vi "2_ExportDatatoExcel.vi"(8 "error in (no error)":errorcluster, 10 "Waveform Graph":waveform(dbl)[](graph), 11 "file path (IN)":path) -> (0 "error out":errorcluster, 3 "file path (OUT)":path)   [LabVIEW 2020]
uses:
  <vilib>/Utility/file.llb/Write Delimited Spreadsheet (string).vi
panel:
  out "Ch3 : Y":dbl[](array[numeric])
  out "Ch3 : appended array":string[](array[string])
  out "Ch1 : appended array":string[](array[string])
  out "Ch1 : Y":dbl[](array[numeric])
  out "dt":dbl
  out "Spread Sheet Display":string[][](array[string])
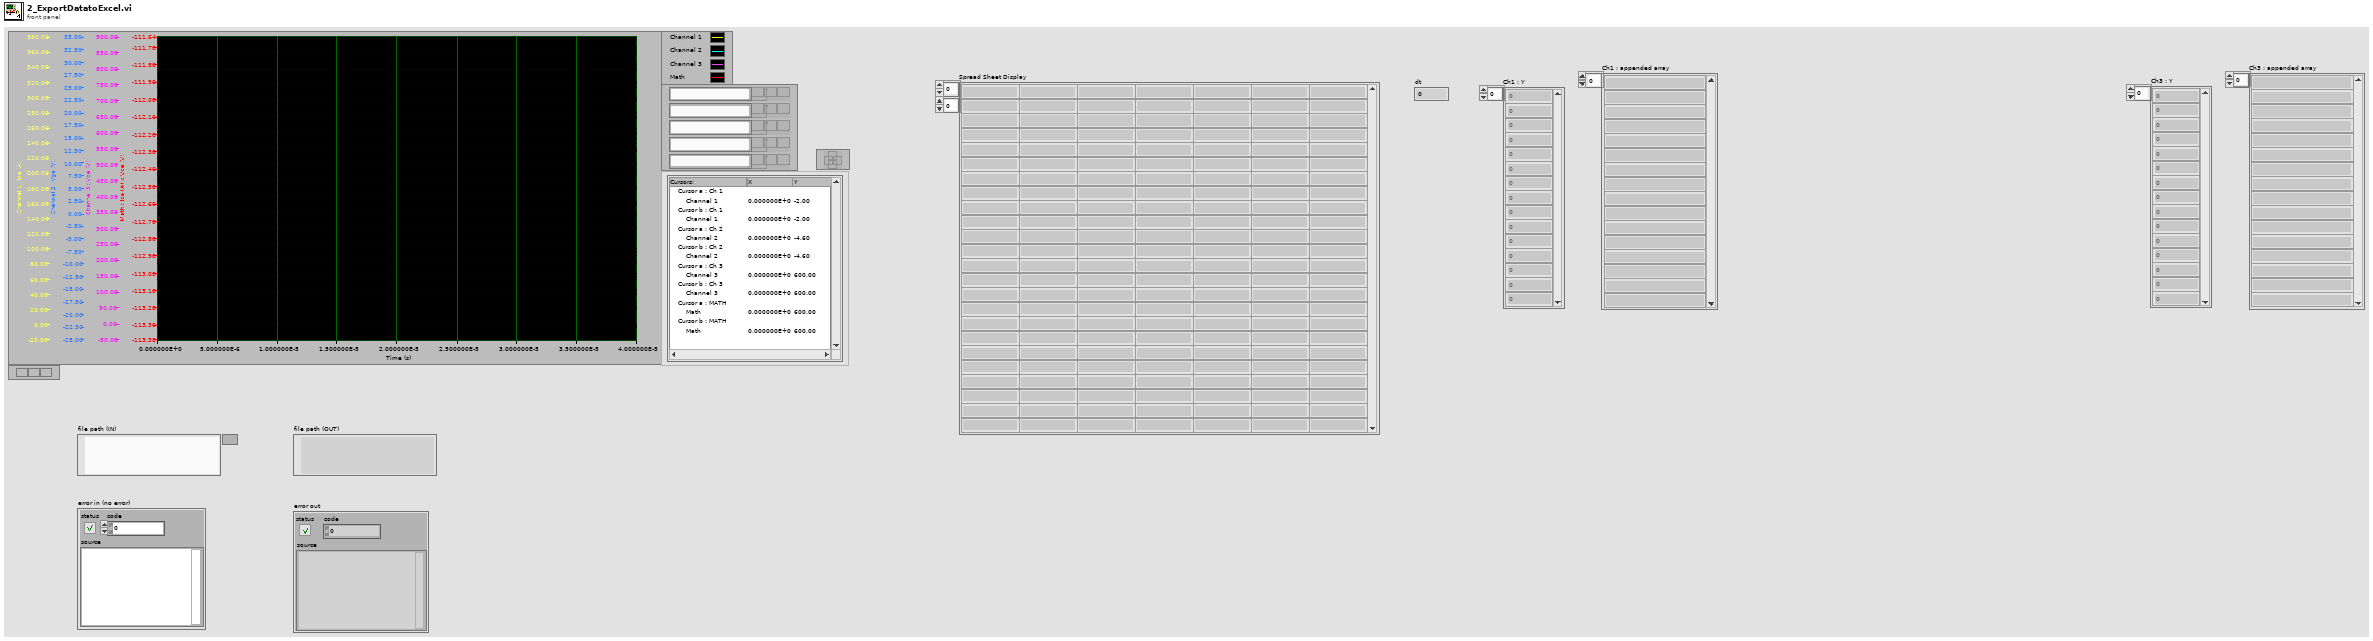
[diagram p1: front panel]
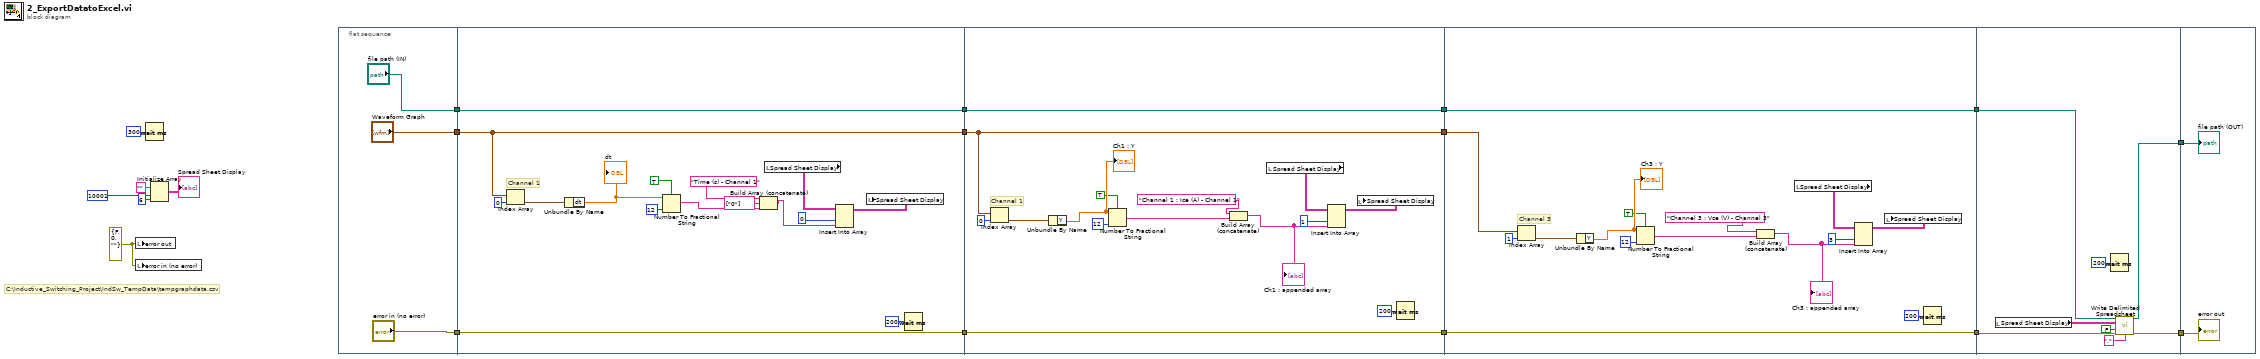
[diagram p0: block diagram]
diagram:
  w8 = errorcluster {"status"=FALSE, "code"=0, "source"=""} ("error out")
  # "C:\\Inductive_Switching_Project\\IndSw_TempData\\tempgraphdata.csv"
  n1 = local write "error out"(w8) -> ()
  n2 = local write "error in (no error)"(w8) -> ()
  n3 = Wait (ms)(milliseconds to wait=u32 300) -> ()  [unwired: 1 out]
  n4 = Initialize Array("", 10001 ("dimension size"), 6 ("dimension size")) -> (→"Spread Sheet Display":string[][])
  n5 = flat-sequence {
    tunnel: ["Waveform Graph"] -> w12
    tunnel: ["error in (no error)"] -> w10
    tunnel: ["file path (IN)"] -> w5
    tunnel: [w26] -> w14
    tunnel: w12 -> [w26]
    tunnel: w10 -> [w25]
    tunnel: [w25] -> w9
    tunnel: [w23] -> w6
    tunnel: w5 -> [w23]
    tunnel: w14 -> [w39]
    tunnel: [w42] -> w3
    tunnel: w9 -> [w42]
    tunnel: [w40] -> w2
    tunnel: w6 -> [w40]
    tunnel: [w39] -> w1
    tunnel: [w57] -> w11
    tunnel: w3 -> [w57]
    tunnel: [w55] -> w7
    tunnel: w2 -> [w55]
    tunnel: w1 -> [w54]
    tunnel: [w73] -> w13
    tunnel: w11 -> [w72]
    tunnel: w7 -> [w70]
    tunnel: [w69] -> w4
    tunnel: w13 -> [w78]
    tunnel: w4 -> [w77]
    frame #0 {
    }
    frame #1 {
      # "Channel 1"
      n6 = Index Array(array=w26, index=0) -> (element=w37:waveform(dbl))
      n7 = Unbundle By Name(w37) -> ("dt"=w35:dbl)
      "dt" <- w35
      n8 = Number To Fractional String(use system decimal point (T)=TRUE, number=w35, precision (6)=i16 12) -> (F-format string=w30:string)  [unwired: 1 in]
      n9 = Build Array (concatenate)("Time (s) - Channel 1", string[] ["0"] ("array"), w30) -> (w29:string[])
      n10 = local read "Spread Sheet Display"() -> (w34:string[][])
      n11 = Insert Into Array(array=w34, index (col)=0 ("disabled index (col)"), new element=w29) -> (w38:string[][])  [unwired: 1 in]
      n12 = local write "Spread Sheet Display"(w38) -> ()
      n13 = Wait (ms)(milliseconds to wait=u32 200) -> ()  [unwired: 1 out]
    }
    frame #2 {
      # "Channel 1"
      n14 = Index Array(array=w39, index=0) -> (element=w49:waveform(dbl))
      n15 = Unbundle By Name(w49) -> ("Y"=w50:dbl[])
      "Ch1 : Y" <- w50
      n16 = Number To Fractional String(use system decimal point (T)=TRUE, number=w50, precision (6)=i16 12) -> (F-format string=w52:string[])  [unwired: 1 in]
      n17 = Build Array (concatenate)("Channel 1 : Ice (A) - Channel 1", w52) -> (w53:string[])
      "Ch1 : appended array" <- w53
      n18 = local read "Spread Sheet Display"() -> (w51:string[][])
      n19 = Insert Into Array(array=w51, index (col)=1 ("disabled index (col)"), new element=w53) -> (w48:string[][])  [unwired: 1 in]
      n20 = local write "Spread Sheet Display"(w48) -> ()
      n21 = Wait (ms)(milliseconds to wait=u32 200) -> ()  [unwired: 1 out]
    }
    frame #3 {
      # "Channel 3"
      n22 = Index Array(array=w54, index=1) -> (element=w64:waveform(dbl))
      n23 = Unbundle By Name(w64) -> ("Y"=w65:dbl[])
      "Ch3 : Y" <- w65
      n24 = Number To Fractional String(use system decimal point (T)=TRUE, number=w65, precision (6)=i16 12) -> (F-format string=w67:string[])  [unwired: 1 in]
      n25 = Build Array (concatenate)("Channel 3 : Vce (V) - Channel 3", w67) -> (w68:string[])
      "Ch3 : appended array" <- w68
      n26 = local read "Spread Sheet Display"() -> (w66:string[][])
      n27 = Insert Into Array(array=w66, index (col)=3 ("disabled index (col)"), new element=w68) -> (w63:string[][])  [unwired: 1 in]
      n28 = local write "Spread Sheet Display"(w63) -> ()
      n29 = Wait (ms)(milliseconds to wait=u32 200) -> ()  [unwired: 1 out]
    }
    frame #4 {
      n30 = local read "Spread Sheet Display"() -> (w76:string[][])
      n31 = Wait (ms)(milliseconds to wait=u32 200) -> ()  [unwired: 1 out]
      n32 = call-poly <vilib>:"Write Delimited Spreadsheet.vi"("file path (dialog if empty)"=w70, "2D data"=w76, "append to file? (new file:F)"=FALSE, "error in (no error)"=w72, "delimiter (\\t)"="," ("delimiter (\\t)")) -> ("new file path (Not A Path if cancelled)"=w69:path, "error out"=w73:errorcluster)  [unwired: 9 in]
    }
    frame #5 {
      "error out" <- w78
      "file path (OUT)" <- w77
    }
  }
